vi "Write State_.vi"(10 "State:":T1, 11 "Model in":refnum<class "Model.lvclass">) -> (3 "Model out":refnum<class "Model.lvclass">)   [LabVIEW 2013, in "Model.lvclass"]
uses:
  Model.lvclass
  Typedefs/StateSelector.ctl
  Model.lvclass/Model.ctl
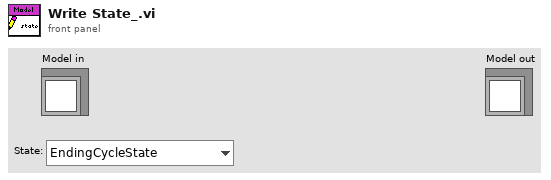
[diagram p1: front panel]
types:
  T1 = typedef "StateSelector.ctl" = enum16{"EndingCycleState", "FaultState", "InteractiveMotionState", "MovingToNewForceState", "OffState", "PausingState", "StandbyState", "StoppedState"}
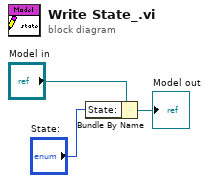
[diagram p0: block diagram]
diagram:
  n1 = Bundle By Name(cluster="Model in", "State:"="State:") -> (→"Model out":refnum<class "Model.lvclass">)
